vi "Unit Delay (DBL Array).vi"(2 "initialize":bool, 3 "initial conditions":dbl[](array[numeric]) format="%.2f", 5 "input points":dbl[](array[numeric]) format="%.2f") -> (1 "output points":dbl[](array[numeric]) format="%.2f")   [LabVIEW 2017, in "NI_AdvCtrl_discrete linear.lvlib"]
doc: "LabVIEW no longer supports this VI. You can obtain similar functionality by installing the LabVIEW Simulation Module.\n\nDelays the input exactly one time step, i.e. output[n]=input[n-1], where output[0]=initial condition."
uses:
  <vilib>/addons/control/advanced/NI_AdvCtrl_discrete linear.lvlib
  <vilib>/addons/control/advanced/NI_AdvCtrl_continuous linear.lvlib
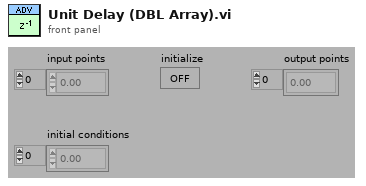
[diagram p1: front panel]
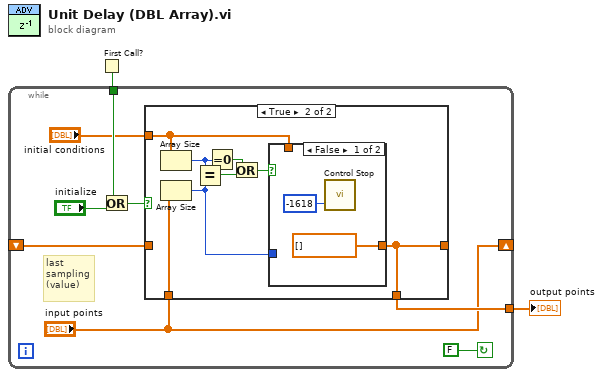
[diagram p0: block diagram]
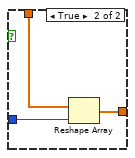
[diagram p3: hidden frame]
diagram:
  n1 = First Call?() -> (First Call?: T/F=w2:bool)
  n2 = while {
    tunnel: w2 -> [w7]
    tunnel: [w9] -> w1
    shift-left: _ -> [w10]
    shift-right: ["input points"] -> _
    stop <- FALSE continue-if-true
    # "last\nsampling\n(value)"
    n3 = Or(x=w7, y="initialize") -> (x .or. y?=w6:bool)
    n4 = case shown="True" w6 {
      tunnel: [w12 w20] -> _
      tunnel: "input points" -> [w12 w18]
      tunnel: [w11 w20] -> w9
      tunnel: w10 -> [w11 _]
      tunnel: "initial conditions" -> [_ w19]
      frame False {
      }
      frame True {
        n5 = Array Size(array=w19) -> (size(s)=w16:i32)
        n6 = Array Size(array=w18) -> (size(s)=w13:i32)
        n7 = Equal?(x=w16, y=w13) -> (x = y?=w17:bool)
        n8 = Equal To 0?(x=w16) -> (x = 0?=w14:bool)
        n9 = Or(x=w14, y=w17) -> (x .or. y?=w15:bool)
        n10 = case shown="False" w15 {
          tunnel: [dbl[] [] ("Initial Conditions") w25] -> w20
          tunnel: w19 -> [_ w24]
          tunnel: w13 -> [_ w23]
          frame False {
            n11 = call <vilib>:"Control Stop.vi"("error"=-1618) -> ()  [unwired: 2 out]
          }
          frame True {
            n12 = Reshape Array(w24, w23) -> (w25:dbl[])
          }
        }
      }
    }
  }
  "output points" <- w1
